vi "Get Job Sequence.vi"(10 "Job Sequence Tree Reference in":refnum<vi>) -> (2 "JOB  Sequence Array":T1(array[cluster]), 3 "Job Sequence Tree Reference out":refnum<vi>)   [LabVIEW 2021]
panel:
  # "EP_JOB - Elevator Positioning\nCSM_JOB - Constant Speed Movement\nSSR_JOB - Staircase Shear Ramp\nLSR_JOB - Linear/Log Shear Ramp"
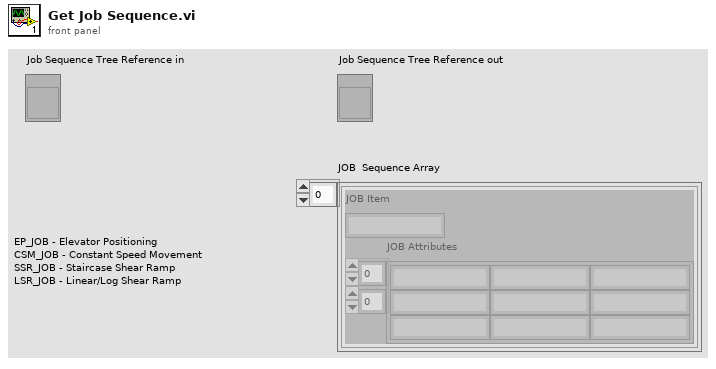
[diagram p1: front panel]
types:
  T1 = cluster{"JOB Item":string, "JOB Attributes":string[][]}[]
  T2 = cluster{"Navigate Tree:Get Child":string, string[][]}
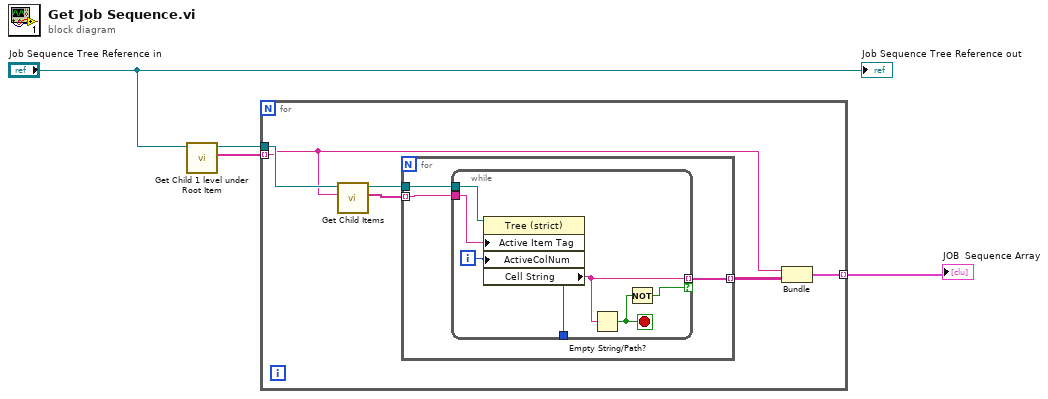
[diagram p0: block diagram]
diagram:
  n1 = call "Get Child 1 level under Root Item.vi"("TreeControl in"="Job Sequence Tree Reference in") -> ("All Child under Root"=w2:string[], "TreeControl out"=w3:refnum<vi>)  [unwired: 9 in]
  n2 = for {
    tunnel: w3 -> [w7]
    tunnel: [w8] -> w1 mode=indexing
    tunnel: w2 -> [w5] mode=indexing
    n3 = call "Get Child Items.vi"("Node"=w5, "TreeControl in"=w7) -> ("Child Array"=w6:string[], "TreeControl out"=w10:refnum<vi>)  [unwired: 8 in]
    n4 = for {
      tunnel: w10 -> [w14]
      tunnel: [w12] -> w9 mode=indexing
      tunnel: w6 -> [w11] mode=indexing
      i -> [w13]
      n5 = while {
        tunnel: w14 -> [w16]
        tunnel: w13 -> [_]
        tunnel: [w19] -> w12 mode=indexing if=w17
        tunnel: w11 -> [w15]
        i -> [w20]
        stop <- w18 stop-if-true
        n6 = property on="Property Node" class="Tree (strict)"(reference=w16, "Active Item Tag"=w15, "ActiveColNum"=w20) -> ("Cell String"=w19:string)  [unwired: 1 in, 2 out]
        n7 = Empty String/Path?(string/path=w19) -> (empty?=w18:bool)
        n8 = Not(x=w18) -> (.not. x?=w17:bool)
      }
    }
    n9 = Bundle("Navigate Tree:Get Child"=w5, w9) -> (w8:T2)  [unwired: 1 in]
  }
  "JOB  Sequence Array" <- w1
  "Job Sequence Tree Reference out" <- "Job Sequence Tree Reference in"
